vi "Global.vi"() -> ()   [LabVIEW 2013]
uses:
  <vilib>/userdefined/High Color/IMAQdx.ctl
  <vilib>/Utility/miscctls.llb/LVAllMonitorsDisplayTypeDef.ctl
  <vilib>/Utility/miscctls.llb/LVRectTypeDef.ctl
panel:
  in  "Reverse Z?":bool caption="Reverse Z"
  in  "Reverse Y?":bool caption="Reverse Y"
  in  "Reverse X?":bool caption="Reverse X"
  out "Stationary?":bool caption="Image Composite?"
  in  "Stationary Count":i32
  out "XYZ LiveS":dbl[](array[numeric]) caption="XYZ Live"
  in  "Review Obj XYZ":dbl[][](array[numeric]) caption="Ref XYZ0"
  out "Review T/F":bool
  in  "Review Obj XYZ in":dbl[][](array[numeric]) caption="Ref XYZ0"
  in  "Review Ref XYZ in":dbl[][](array[numeric]) caption="Ref XYZ0"
  in  "ZOffset Light":dbl[](array[numeric])
  in  "Test Numeric Array":dbl[][](array[numeric])
  in  "Focus Fraction":dbl=0.5
  out "Focus Quality":dbl
  in  "Home Pattern XYZ":dbl[][][](array[numeric])
  in  "Home WH":dbl[][][](array[numeric])
  in  "Home Increment":dbl
  out "Home Pattern":T1[][](array[plugin-control])
  in  "Z-AXIS_KD":string="0"
  in  "Z-AXIS_KI":string="10"
  in  "Z-AXIS_KP":string="1000"
  in  "Z-AXIS_PCROS":string="0.000055"
  in  "Cursor Optics":i32
  in  "Obj XYZ1 Optics":dbl[][](array[numeric])
  in  "Obj XYZ0 Optics":dbl[][](array[numeric])
  out "Sample Data Write?":bool=TRUE
  in  "Sample Data Queue":string[][](array[string])
  in  "XYZdZ":dbl[](array[numeric])
  in  "dZ_sign":dbl=1.0
  out "Refined?":bool
  out "Skip?":bool
  in  "Pi":dbl=3.14159
  out "Add Number?":bool
  out "Add Loop?":bool
  out "XYZ Active?":bool
  in  "Z RIndex":dbl
  in  "Test String Array":string[][](array[string])
  in  "Obj1 Ref Index":i32=-1
  in  "Obj1 Index Max":i32=-1
  in  "Obj1":string[](array[string])
  in  "Obj SD XYZ1":string[][][](array[string])
  out "Ref T/F Transform":bool
  in  "Obj0 Ref Index":i32=-1
  in  "Obj0 Index Max":i32=-1
  in  "Obj SD XYZ0":string[][][](array[string])
  in  "Obj Number":i32=-1
  in  "OBJ_Description":string[][](array[string])
  in  "Obj Index":i32=-1
  in  "Obj Label XYZ1":string[][](array[string])
  in  "Obj Label XYZ0":string[][](array[string])
  in  "Obj XYZ1":dbl[][][](array[numeric])
  in  "Obj XYZ0":dbl[][][](array[numeric])
  in  "Obj Points XYZ1":i32[](array[numeric])
  in  "Obj Points XYZ0":i32[](array[numeric])
  in  "Obj0":string[](array[string])
  in  "Skip to Index":i32
  out "Skip To":bool
  in  "Ref Optics Index":i32
  in  "Z-AXIS bytes":u32=40
  in  "XY-STAGE bytes":u32=70
  in  "Z Fine instr":dbl
  in  "VI Name Active":string
  in  "Comp Image Optics Index":i32=1
  in  "Microscope Magnification":dbl[](array[numeric])
  in  "Z-AXIS maskT":u16=128
  in  "XY-STAGE maskT":u16=128
  out "Smart Refine":bool=TRUE
  in  "ZOffset Objective":dbl[](array[numeric])
  in  "YOffset Objective":dbl[](array[numeric])
  in  "XOffset Objective":dbl[](array[numeric])
  in  "Vision Folder":path=path "C:/A2Z/Projects"
  out "XYZ Live":dbl[](array[numeric])
  out "RefreshTo":dbl
  in  "RefreshPeriod":dbl=200000.0
  in  "Sample Data in":string[][](array[string])
  in  "FP:POffset":T2
  in  "FP:WOffset":T3
  out "Live_Raw":T1(plugin-control)
  out "Display:Primary Workspace":T4
  out "Display:All Monitors":T5
  in  "Filename Root O/S":string[](array[string])
  in  "Microscope Light Index":i32=1
  in  "Microscope Optics Index":i32=3
  in  "Microscope Light":string[](array[string])
  in  "Microscope Optics":string[](array[string])
  in  "Image Height":dbl[](array[numeric])
  in  "Image Width":dbl[](array[numeric])
  in  "max VI":i32=10
  in  "min VI":i32=5
  in  "Operation Target":string
  out "Image NULL":T1(plugin-control)
  in  "Operation Mode":string="New/Append"
  in  "VI Menu Refnum":refnum<k9>[](array[refnum])
  in  "VI Menu":string[](array[string])=["XYZStage.vi:USER_", ""]
  in  "Y Micron/Pixel HP":dbl
  in  "X Micron/Pixel HP":dbl
  out "Append":bool
  in  "OS Reentrant Index":i32
  in  "IMAQdx Session":T6="cam4"
  in  "user event reg refnum_Boolean":refnum<event-registration>[](array[refnum])
  in  "user event name_Boolean":string[](array[string])=["XYZStage_Language.vi:Boolean0", "Operate_XYZ.vi:Boolean0", "Operate_Keyboard.vi:Boolean0", "Vision_Autofocus.vi:Boolean0", "Vision_AVI.vi:Boolean0", "View_Data.vi:Boolean0", "View_Profile.vi:Boolean0", "Vision_Live.vi:Boolean0", "Vision_Sample_Map.vi:Boolean0"]
  in  "user event out_Boolean":refnum<user-event>[](array[refnum])
  in  "Ref Points Count XYZ1":i32=-1
  out "Live":bool=TRUE
  in  "Ref Best XYZ1":dbl[][](array[numeric])
  in  "Ref Best XYZ0":dbl[][](array[numeric])
  in  "Ref XYZ1":dbl[][](array[numeric])
  in  "Ref XYZ0":dbl[][](array[numeric])
  in  "Ref Label XYZ1":string[](array[string])
  in  "Ref Label XYZ0":string[](array[string])
  out "Script CS":bool[](array[boolean])
  in  "Loop Index":i32[](array[numeric])
  in  "OP_Description":string[][](array[string])
  in  "VISA":refnum<visa-resource-name>[](array[refnum])=["COM1", "COM2", "COM3", "COM4", "COM5", "COM6", "COM7", "COM8", "COM9"]
  in  "Sample Data":string[][](array[string])
  in  "XYZStage Execution Disk":path
  in  "Z-AXIS item tag":string[](array[string])
  in  "XY-STAGE item tag":string[](array[string])
  in  "Z-AXIS expected reply":string[](array[string])
  in  "Z-AXIS command":string[](array[string])
  in  "Z-AXIS reply terminator":string="\r\n"
  in  "Z-AXIS termination char\n(0xA = '\\n' = LF)":u8=13
  in  "Z-AXIS command terminator":string="\r"
  in  "Z-AXIS mask":u16=64
  in  "Z-AXIS VISA resource name":refnum<visa-resource-name>="COM4"
  in  "Z-AXIS stop bits":u16(ring)=10 items=["1.0"=10, "1.5"=15, "2.0"=20]
  in  "Z-AXIS flow control":u16(ring) items=["None", "XON/XOFF", "RTS/CTS", "XON/XOFF & RTS/CTS", "DTR/DSR", "XON/XOFF & DTR/DSR"]
  in  "Z-AXIS parity":enum16{"None", "Odd", "Even", "Mark", "Space"}(ring)
  in  "Z-AXIS data bits":u16=8
  in  "Z-AXIS baud rate":u32=9600
  in  "XY-STAGE expected reply":string[](array[string])
  in  "XY-STAGE command":string[](array[string])
  in  "XY-STAGE reply terminator":string="\n"
  in  "XY-STAGE termination char\n(0xA = '\\n' = LF)":u8=13
  in  "XY-STAGE command terminator":string="\r"
  in  "XY-STAGE mask":u16=64
  in  "XY-STAGE VISA resource name":refnum<visa-resource-name>="COM10"
  in  "XY-STAGE stop bits":u16(ring)=20 items=["1.0"=10, "1.5"=15, "2.0"=20]
  in  "XY-STAGE flow control":u16(ring) items=["None", "XON/XOFF", "RTS/CTS", "XON/XOFF & RTS/CTS", "DTR/DSR", "XON/XOFF & DTR/DSR"]
  in  "XY-STAGE parity":enum16{"None", "Odd", "Even", "Mark", "Space"}(ring)
  in  "XY-STAGE data bits":u16=8
  in  "XY-STAGE baud rate":u32=9600
  in  "Ref Points In XYZ0":i32=-1
  in  "Ref Points XYZ0":i32=-1
  out "Ref T/F XYZ1":bool[](array[boolean])
  in  "Script Completed Max":i32=-1
  in  "Script Line Rank":i32[](array[numeric])
  in  "Script Completed":i32[](array[numeric])=[-1]
  in  "Script Events":i32
  in  "Script Loop Rank":i32=-1
  in  "Script":string[][](array[string])=[[""]]
  in  "Script Run Rank":i32
  in  "VI RefNum":refnum<vi>[](array[refnum])
  in  "FP:Title":string[](array[string])
  out "FP:Personalize":bool[](array[boolean])
  in  "FP:Origin":cluster{"Horizontal":i16[], "Vertical":i16[]}={"Horizontal"=[0], "Vertical"=[0]}
  in  "FP:Panel.Bounds":T7={"Left"=[0], "Top"=[0], "Right"=[0], "Bottom"=[0]}
  in  "FP:Window.Bounds":T7={"Left"=[0], "Top"=[0], "Right"=[0], "Bottom"=[0]}
  in  "FP:Monitor":u16[](array[numeric])=[0]
  in  "VI":string[](array[string])=["XYZStage.vi", "XYZStage_Language.vi", "Vision_Sample_Map.vi", "Operate_Script_Reentrant.vi", "Operate_Script.vi", "Operate_XYZ.vi", "Operate_Keyboard.vi", "Vision_Autofocus.vi", "Vision_AVI.vi", "View_Data.vi", "View_Profile.vi", "Vision_Live.vi", "XYZ_Transformation_Setup.vi", "XYZ_Transformation_Math.vi", "Operate_Measure.vi", "XYZ_XYStage.vi", "XYZ_ZAxis.vi", "Operate_XYZ_Event_TC.vi", "Operate_XYZ_Remote.vi", "XYZ_dZ.vi", "Vision_Pattern.vi", "Message_Pause.vi", "XY_Graph.vi", "Vision_AVI_Manual.vi", "Scan_Area.vi", "XYZ_Optics_Calibrate.vi"]
  in  "VI Refnum Active":refnum<vi>
  in  "Language Index":i32
  in  "Recent Script  File":path=path "Scripts/XYZStage_Script_Recent.txt" caption="Recent Profile Path"
  in  "Recent Profile File":path=path "Profiles/XYZStage_Profile_Recent.txt" caption="Recent Profile Path"
  in  "Recent XYZStage Execution Folder":path=path "C:/XYZStage"
  in  "Language Item English":string[](array[string])=[""]
  out "Analyst":string
  out "Analysis":string
  out "Label":string
  out "Material":string
  out "Sample":string
  out "Project":string
  in  "Write File":string
  in  "Write Folder":path
  in  "Script File":path=path "Scripts/XYZStage_Script_Default.txt" caption="Script Path"
  in  "Profile File":path=path "Profiles/XYZStage_Profile_Default.txt" caption="Profile Path"
  in  "XYZStage Execution Folder":path=path "C:/XYZStage"
  in  "Profile Item User Language":string[](array[string])=[""]
  in  "Profile Item English(US)":string[](array[string])=[""]
  in  "Profile Item Value":string[](array[string])=[""]
  in  "Profile Item Tag":string[](array[string])=[""]
  in  "Language Language Name":string[](array[string])=[""]
  in  "Language Item User Language":string[](array[string])=[""]
  in  "Language Item Tag":string[](array[string])=[""]
  # "Selected Path Settings"
  # "Recent  Path Settings"
  # "Profile"
  # "Script"
  # "XY-STAGE VISA"
  # "Z-AXIS VISA"
  # "Camera IMAQdx"
  # "Sample Data"
  # "OPERATION and OBJECT"
  # "VISA Configuration"
  # "VISA Configuration"
  # "Sample Identification"
  # "ASI com4\nLudl com9"
  # "Microscope"
  # "ASI 1.0 stop  bits\nLudl 2.0 stolp bits"
  # "XYZ"
  # "Display"
  # "VISA Flush Buffer"
  # "VISA Flush Buffer"
  # "REFERENCE"
  # "ASI \\r\nLudl \\r"
  # "\\r\\n"
  # "ASI \\r\\n\nLudl \\n"
  # "\\r"
  # "OBJECT"
  # "Optiphot2 0.000001\nEcliplse 0.000055"
  # "Optipho2 1500\nEclipse 300"
  # "Optiphot2 5\nEclipse 20"
  # "Optiphot2 0\nEclipse 0"
  # "XYZ Position Correction"
  # "optics\nobject\nxyz"
  # "optics\nobject"
  # "optics\nobject\nwh"
  # "Script Loop Rank\nScript Loop Index(rank)"
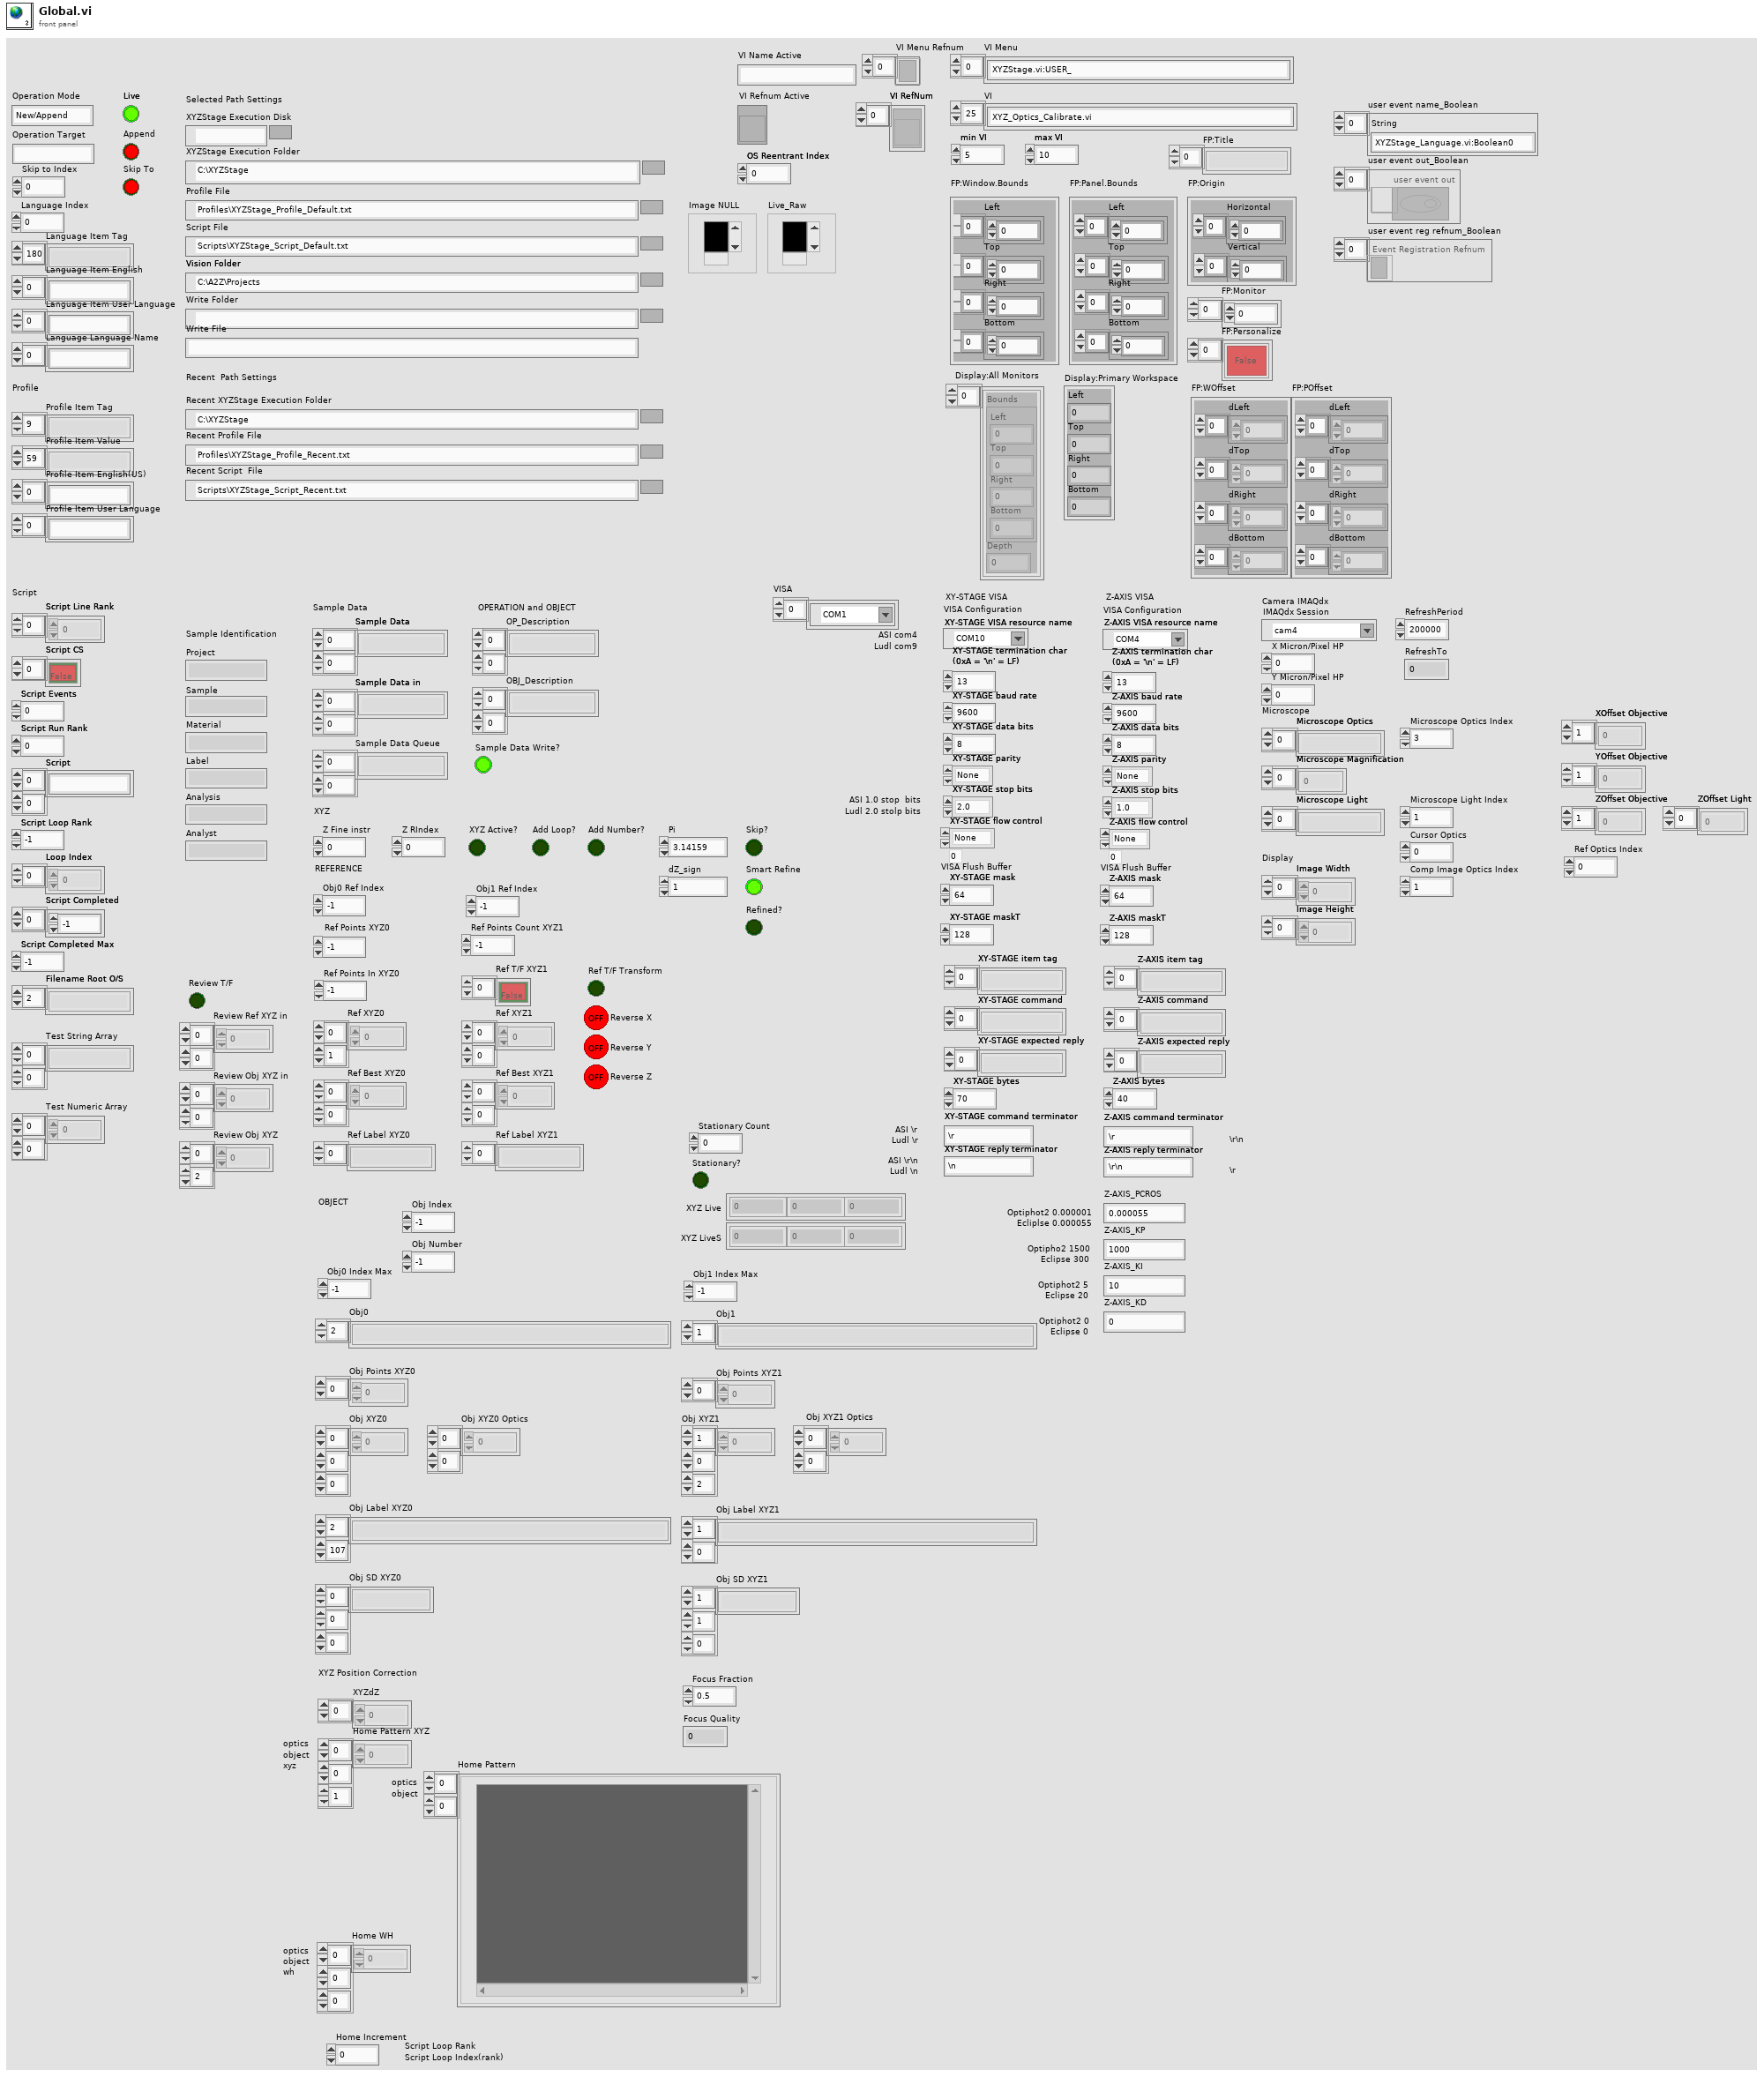
[diagram p1: front panel]
types:
  T1 = typedef "IMAQ Image.ctl" = refnum<image>
  T2 = cluster{"dLeft":i16[], "dTop":i16[], "dRight":i16[], "dBottom":i16[]}
  T3 = cluster{"dLeft":i16[], "dTop":i16[], "dRight":i32[], "dBottom":i16[]}
  T4 = typedef "LVRectTypeDef.ctl" = cluster{"Left":i16, "Top":i16, "Right":i16, "Bottom":i16}
  T5 = typedef "LVAllMonitorsDisplayTypeDef.ctl" = cluster{"Bounds":cluster{"Left":i16, "Top":i16, "Right":i16, "Bottom":i16}, "Depth":i16}[]
  T6 = typedef "IMAQdx.ctl" = refnum<k21>
  T7 = cluster{"Left":i16[], "Top":i16[], "Right":i16[], "Bottom":i16[]}
diagram:
